vi "StartTrial.vi"(8 "error in (no error)":errorcluster, 11 "TrialBasedExperiment in":refnum<class "DotMappingExperiment.lvclass">) -> (0 "error out":errorcluster, 3 "TrialBasedExperiment out":refnum<class "DotMappingExperiment.lvclass">)   [LabVIEW 2010]
uses:
  DotMappingExperiment.lvclass
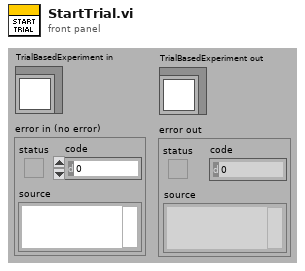
[diagram p1: front panel]
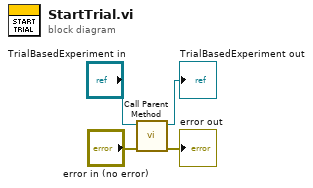
[diagram p0: block diagram]
diagram:
  n1 = call-parent "Call Parent Method"("error in (no error)"="error in (no error)", "TrialBasedExperiment in"="TrialBasedExperiment in") -> ("error out"=→"error out":errorcluster, "TrialBasedExperiment out"=→"TrialBasedExperiment out":refnum<class "DotMappingExperiment.lvclass">)  [unwired: 8 in]
